vi "Config - validate.vi"(8 "error in (no error)":errorcluster) -> (0 "error out":errorcluster)   [LabVIEW 2026, in "Tests.lvlib"]
doc: "Unit test (Caraya) for launch-config validation.\nDrives each pure DTO validator with a deliberately bad field and asserts the specific Lumberjack error code, then drives valid inputs and asserts no error: schemaVersion membership (5021), bounded queueBound/maxFileSize/maxFileCount (5022), routed level range order (5023), empty appender id (5024), and filesystem-safe baseName/extension (5020).\nPure test: builds DTO cluster constants and calls the validators directly. Each fault case captures and clears its expected error so the assert chain is not poisoned. No actors, no file I/O.\n\nImplements LMBR-T-024, T-026, T-027 -> SRS-048, SRS-033/034/056. Assert-level IDs: Test-ID-Assert-Checklist.md."
uses:
  Tests.lvlib
  src/TypeDefs/ConfigDTO/AppenderConfigDTO.ctl
  src/TypeDefs/ConfigDTO/FilterDTO.ctl
  src/TypeDefs/ConfigDTO/FileConfigDTO.ctl
  <vilib>/addons/_JKI Toolkits/Caraya/classes/Assert/Assert Not Error.vi
  <vilib>/addons/_JKI Toolkits/Caraya/classes/Assert/Assert Error.vi
  <vilib>/addons/_JKI Toolkits/Caraya/classes/Test/Test.lvclass
  src/Lumberjack.lvlib
  <vilib>/addons/_JKI Toolkits/Caraya/classes/Assert/Assert.lvclass
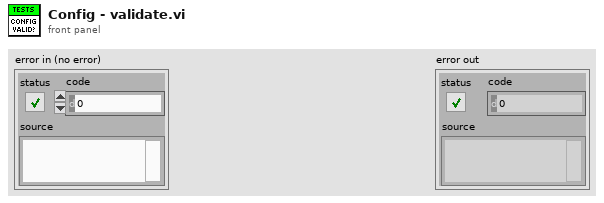
[diagram p1: front panel]
types:
  T1 = typedef "Lumberjack.lvlib/FilterDTO.ctl" = cluster{"mode":string, "levelMin":string, "levelMax":string, "tagPrefix":string}
  T2 = typedef "Lumberjack.lvlib/FileConfigDTO.ctl" = cluster{"rootFolder":string, "maxFileSize":i64, "maxFileCount":i32, "baseName":string, "extension":string, "delimiter":string, "calendarFolderTree":bool}
  T3 = typedef "Lumberjack.lvlib/AppenderConfigDTO.ctl" = cluster{"id":string, "threshold":string, "filter":T1, "queueBound":i32, "dropPolicy":string, "useUTC":bool}
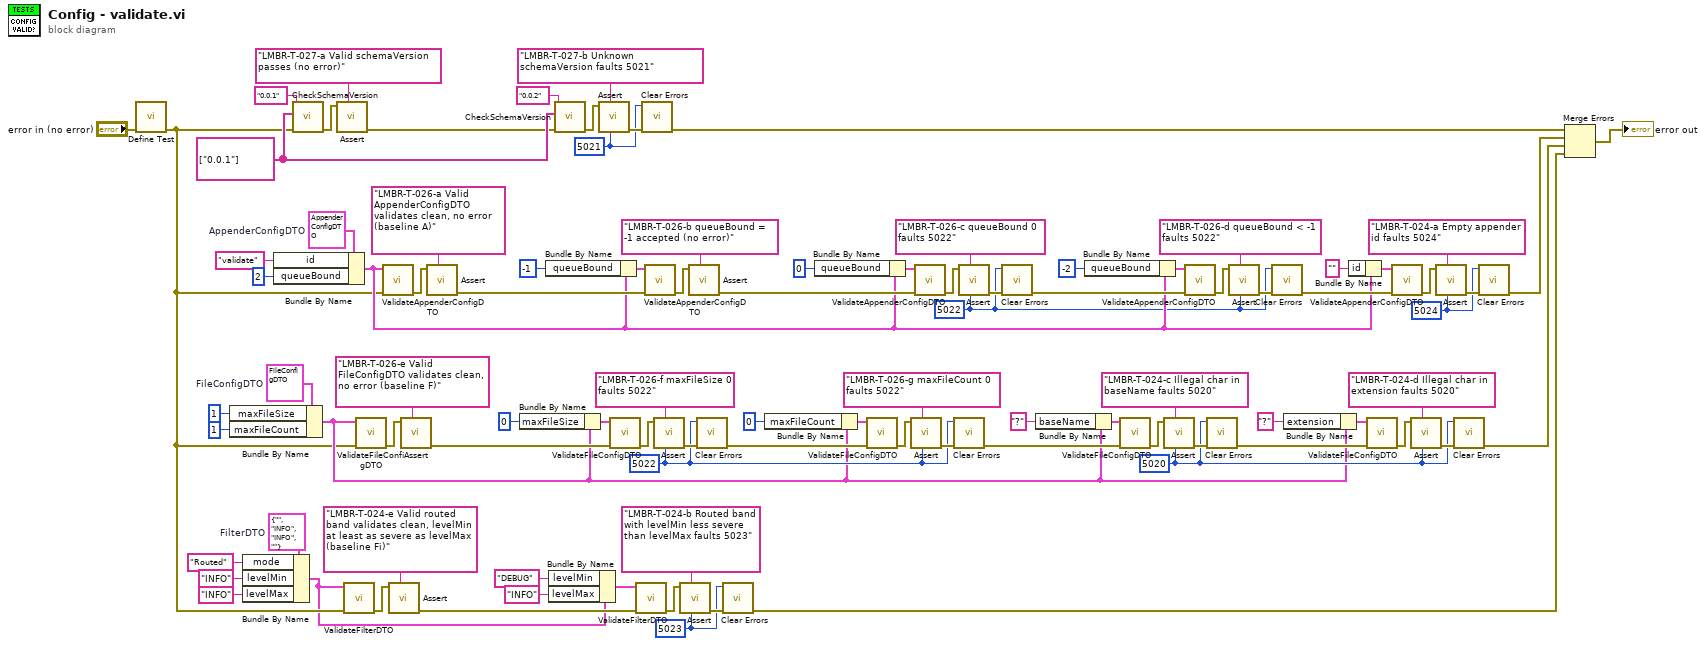
[diagram p0: block diagram]
diagram:
  w7 = 5023 ("error code (1)")
  w17 = T1 {"mode"="", "levelMin"="INFO", "levelMax"="INFO", "tagPrefix"=""}  # FilterDTO
  w20 = 5020 ("error code (1)")
  w33 = 5022 ("error code (1)")
  w65 = T2 {"rootFolder"="", "maxFileSize"=0, "maxFileCount"=0, "baseName"="", "extension"="DropOldest", "delimiter"="", "calendarFolderTree"=FALSE}  # FileConfigDTO
  w38 = 5024 ("error code (1)")
  w35 = 5022 ("error code (1)")
  w81 = T3 {"id"="", "threshold"="INFO", "filter"={"mode"="Mirror", "levelMin"="INFO", "levelMax"="INFO", "tagPrefix"=""}, "queueBound"=0, "dropPolicy"="DropOldest", "useUTC"=FALSE}  # AppenderConfigDTO
  w40 = 5021 ("error code (1)")
  w91 = string[] ["0.0.1"] ("ValidSchemaVersions")
  n1 = call <vilib>:"Define Test.vi"("error in (no error)"="error in (no error)") -> ("error out"=w14:errorcluster)  [unwired: 9 in, 1 out]
  n2 = Bundle By Name(cluster=w65, "maxFileSize"=i64 1 ("queueBound"), "maxFileCount"=1) -> (w19:T2)
  n3 = Bundle By Name(cluster=w17, "mode"="Routed", "levelMin"="INFO", "levelMax"="INFO") -> (w4:T1)
  n4 = Bundle By Name(cluster=w81, "id"="validate", "queueBound"=2) -> (w37:T3)
  n5 = call "CheckSchemaVersion.vi"("error in (no error)"=w14, "ValidSchemaVersions"=w91, "schemaVersionIn"="0.0.1") -> ("error out"=w87:errorcluster)  [unwired: 6 in, 2 out]
  n6 = call-poly <vilib>:"Assert.vi"("Label"="LMBR-T-027-a Valid schemaVersion passes (no error)", "Not Error?"=w87) -> ("error out"=w86:errorcluster)  [unwired: 8 in, 1 out]
  n7 = call "ValidateFilterDTO.vi"("error in (no error)"=w14, "FilterDTOin"=w4) -> ("error out"=w15:errorcluster)  [unwired: 8 in, 1 out]
  n8 = call "ValidateFileConfigDTO.vi"("error in (no error)"=w14, "FileConfigDTOin"=w19) -> ("error out"=w55:errorcluster)  [unwired: 8 in, 1 out]
  n9 = call "ValidateAppenderConfigDTO.vi"("error in (no error)"=w14, "AppenderConfigDTOin"=w37) -> ("error out"=w49:errorcluster)  [unwired: 8 in, 1 out]
  n10 = call-poly <vilib>:"Assert.vi"("Label"="LMBR-T-024-e Valid routed band validates clean, levelMin at least as severe as levelMax (baseline Fi)", "Not Error?"=w15) -> ("error out"=w6:errorcluster)  [unwired: 8 in, 1 out]
  n11 = call-poly <vilib>:"Assert.vi"("Label"="LMBR-T-026-e Valid FileConfigDTO validates clean, no error (baseline F)", "Not Error?"=w55) -> ("error out"=w53:errorcluster)  [unwired: 8 in, 1 out]
  n12 = call-poly <vilib>:"Assert.vi"("Label"="LMBR-T-026-a Valid AppenderConfigDTO validates clean, no error (baseline A)", "Not Error?"=w49) -> ("error out"=w46:errorcluster)  [unwired: 8 in, 1 out]
  n13 = Bundle By Name(cluster=w19, "maxFileSize"=i64 0) -> (w52:T2)
  n14 = Bundle By Name(cluster=w37, "queueBound"=-1) -> (w39:T3)
  n15 = Bundle By Name(cluster=w4, "levelMin"="DEBUG", "levelMax"="INFO") -> (w5:T1)
  n16 = call "CheckSchemaVersion.vi"("error in (no error)"=w86, "ValidSchemaVersions"=w91, "schemaVersionIn"="0.0.2") -> ("error out"=w88:errorcluster)  [unwired: 6 in, 2 out]
  n17 = call-poly <vilib>:"Assert.vi"("error code (1)"=w40, "Label"="LMBR-T-027-b Unknown schemaVersion faults 5021", "Error?"=w88) -> ("error out"=w42:errorcluster)  [unwired: 7 in, 1 out]
  n18 = call "ValidateFileConfigDTO.vi"("error in (no error)"=w53, "FileConfigDTOin"=w52) -> ("error out"=w62:errorcluster)  [unwired: 8 in, 1 out]
  n19 = call "ValidateFilterDTO.vi"("error in (no error)"=w6, "FilterDTOin"=w5) -> ("error out"=w9:errorcluster)  [unwired: 8 in, 1 out]
  n20 = call <vilib>:"Clear Errors.vi"("error in (no error)"=w42, "specific error code to clear (0: all)"=w40) -> ("error out"=w41:errorcluster)  [unwired: 4 in, 1 out]
  n21 = call "ValidateAppenderConfigDTO.vi"("error in (no error)"=w46, "AppenderConfigDTOin"=w39) -> ("error out"=w82:errorcluster)  [unwired: 8 in, 1 out]
  n22 = call-poly <vilib>:"Assert.vi"("error code (1)"=w33, "Label"="LMBR-T-026-f maxFileSize 0 faults 5022", "Error?"=w62) -> ("error out"=w61:errorcluster)  [unwired: 7 in, 1 out]
  n23 = call-poly <vilib>:"Assert.vi"("error code (1)"=w7, "Label"="LMBR-T-024-b Routed band with levelMin less severe than levelMax faults 5023", "Error?"=w9) -> ("error out"=w8:errorcluster)  [unwired: 7 in, 1 out]
  n24 = call-poly <vilib>:"Assert.vi"("Label"="LMBR-T-026-b queueBound = -1 accepted (no error)", "Not Error?"=w82) -> ("error out"=w45:errorcluster)  [unwired: 8 in, 1 out]
  n25 = call <vilib>:"Clear Errors.vi"("error in (no error)"=w61, "specific error code to clear (0: all)"=w33) -> ("error out"=w60:errorcluster)  [unwired: 4 in, 1 out]
  n26 = call <vilib>:"Clear Errors.vi"("error in (no error)"=w8, "specific error code to clear (0: all)"=w7) -> ("error out"=w3:errorcluster)  [unwired: 4 in, 1 out]
  n27 = Bundle By Name(cluster=w19, "maxFileCount"=0) -> (w58:T2)
  n28 = Bundle By Name(cluster=w37, "queueBound"=0) -> (w78:T3)
  n29 = call "ValidateFileConfigDTO.vi"("error in (no error)"=w60, "FileConfigDTOin"=w58) -> ("error out"=w66:errorcluster)  [unwired: 8 in, 1 out]
  n30 = call-poly <vilib>:"Assert.vi"("error code (1)"=w33, "Label"="LMBR-T-026-g maxFileCount 0 faults 5022", "Error?"=w66) -> ("error out"=w34:errorcluster)  [unwired: 7 in, 1 out]
  n31 = call "ValidateAppenderConfigDTO.vi"("error in (no error)"=w45, "AppenderConfigDTOin"=w78) -> ("error out"=w83:errorcluster)  [unwired: 8 in, 1 out]
  n32 = call <vilib>:"Clear Errors.vi"("error in (no error)"=w34, "specific error code to clear (0: all)"=w33) -> ("error out"=w27:errorcluster)  [unwired: 4 in, 1 out]
  n33 = call-poly <vilib>:"Assert.vi"("error code (1)"=w35, "Label"="LMBR-T-026-c queueBound 0 faults 5022", "Error?"=w83) -> ("error out"=w77:errorcluster)  [unwired: 7 in, 1 out]
  n34 = call <vilib>:"Clear Errors.vi"("error in (no error)"=w77, "specific error code to clear (0: all)"=w35) -> ("error out"=w72:errorcluster)  [unwired: 4 in, 1 out]
  n35 = Bundle By Name(cluster=w19, "baseName"="?") -> (w28:T2)
  n36 = Bundle By Name(cluster=w37, "queueBound"=-2) -> (w73:T3)
  n37 = call "ValidateFileConfigDTO.vi"("error in (no error)"=w27, "FileConfigDTOin"=w28) -> ("error out"=w31:errorcluster)  [unwired: 8 in, 1 out]
  n38 = call-poly <vilib>:"Assert.vi"("error code (1)"=w20, "Label"="LMBR-T-024-c Illegal char in baseName faults 5020", "Error?"=w31) -> ("error out"=w30:errorcluster)  [unwired: 7 in, 1 out]
  n39 = call "ValidateAppenderConfigDTO.vi"("error in (no error)"=w72, "AppenderConfigDTOin"=w73) -> ("error out"=w75:errorcluster)  [unwired: 8 in, 1 out]
  n40 = call <vilib>:"Clear Errors.vi"("error in (no error)"=w30, "specific error code to clear (0: all)"=w20) -> ("error out"=w21:errorcluster)  [unwired: 4 in, 1 out]
  n41 = call-poly <vilib>:"Assert.vi"("error code (1)"=w35, "Label"="LMBR-T-026-d queueBound < -1 faults 5022", "Error?"=w75) -> ("error out"=w71:errorcluster)  [unwired: 7 in, 1 out]
  n42 = call <vilib>:"Clear Errors.vi"("error in (no error)"=w71, "specific error code to clear (0: all)"=w35) -> ("error out"=w44:errorcluster)  [unwired: 4 in, 1 out]
  n43 = Bundle By Name(cluster=w19, "extension"="?" ("baseName")) -> (w22:T2)
  n44 = Bundle By Name(cluster=w37, "id"="") -> (w36:T3)
  n45 = call "ValidateFileConfigDTO.vi"("error in (no error)"=w21, "FileConfigDTOin"=w22) -> ("error out"=w25:errorcluster)  [unwired: 8 in, 1 out]
  n46 = call "ValidateAppenderConfigDTO.vi"("error in (no error)"=w44, "AppenderConfigDTOin"=w36) -> ("error out"=w69:errorcluster)  [unwired: 8 in, 1 out]
  n47 = call-poly <vilib>:"Assert.vi"("error code (1)"=w20, "Label"="LMBR-T-024-d Illegal char in extension faults 5020", "Error?"=w25) -> ("error out"=w24:errorcluster)  [unwired: 7 in, 1 out]
  n48 = call-poly <vilib>:"Assert.vi"("error code (1)"=w38, "Label"="LMBR-T-024-a Empty appender id faults 5024", "Error?"=w69) -> ("error out"=w68:errorcluster)  [unwired: 7 in, 1 out]
  n49 = call <vilib>:"Clear Errors.vi"("error in (no error)"=w24, "specific error code to clear (0: all)"=w20) -> ("error out"=w18:errorcluster)  [unwired: 4 in, 1 out]
  n50 = call <vilib>:"Clear Errors.vi"("error in (no error)"=w68, "specific error code to clear (0: all)"=w38) -> ("error out"=w43:errorcluster)  [unwired: 4 in, 1 out]
  n51 = Merge Errors(w41, w43, w18, w3) -> (→"error out":errorcluster)
